vi "Untitled 41.vi"() -> ()   [LabVIEW 2017]
uses:
  driveLogicStates.ctl
panel:
  in  "Boolean 4":bool
  in  "Boolean 3":bool
  in  "Boolean 2":bool
  in  "Boolean":bool
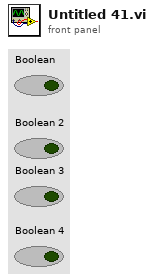
[diagram p1: front panel]
types:
  T1 = typedef "driveLogicStates.ctl" = enum16{"doNothing", "driveDistance", "turnAngle", "freestyle", "guidedDrive", "approachingElement"}
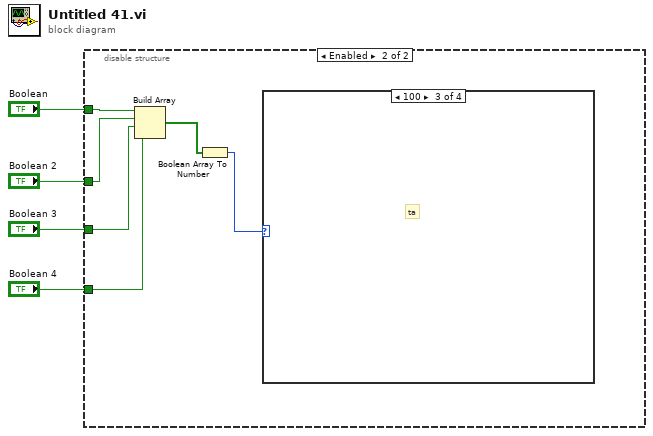
[diagram p0: block diagram]
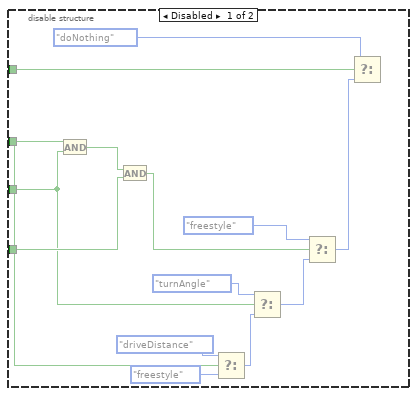
[diagram p2: hidden frame]
diagram:
  n1 = disable-structure shown="Enabled" {
    disable-tunnel: "Boolean" -> [w18 w24]
    disable-tunnel: "Boolean 4" -> [w14 w21]
    disable-tunnel: "Boolean 3" -> [w11 w22]
    disable-tunnel: "Boolean 2" -> [w7 w23]
    frame Disabled {
      n2 = And(x=w7, y=w11) -> (x .and. y?=w13:bool)
      n3 = And(x=w13, y=w14) -> (x .and. y?=w12:bool)
      n4 = Select(t=driveLogicStates."driveDistance", s=w7, f=driveLogicStates."freestyle") -> (s? t:f=w6:T1)
      n5 = Select(t=driveLogicStates."turnAngle", s=w11, f=w6) -> (s? t:f=w9:T1)
      n6 = Select(t=driveLogicStates."freestyle", s=w12, f=w9) -> (s? t:f=w15:T1)
      n7 = Select(t=driveLogicStates."doNothing", s=w18, f=w15) -> ()  [unwired: 1 out]
    }
    frame Enabled {
      n8 = Build Array(w24, w23, w22, w21) -> (w20:bool[])
      n9 = Boolean Array To Number(Boolean array=w20) -> (number=w19:u32)
      n10 = case shown="100" w19 {
        frame 0, 1, 3, 5 {
          # "f"
        }
        frame 8..15, Default {
          # "N"
        }
        frame 4 {
          # "ta"
        }
        frame 2 {
          # "dd"
        }
      }
    }
  }
